vi "VCI_ReadErrInfo.vi"(8 "error in (no error)":errorcluster caption="错误输入（无错误）", 9 "CANIndex":u32, 10 "DevIndex":u32, 11 "DevType":T2=2 items=["USB-CAN"=2, "USB-CAN2"=3]) -> (0 "error out":errorcluster caption="错误输出", 2 "VCI_ERR_INFO":T1, 3 "Return Val":T3=1 items=["OK"=1, "ERROR1"=0, "ERROR2"=-1])   [LabVIEW 2018, in "ControlCan.lvlib"]
uses:
  ControlCan.lvlib
  Return Val.ctl
  DevType.ctl
  VCI_ERR_INFO.ctl
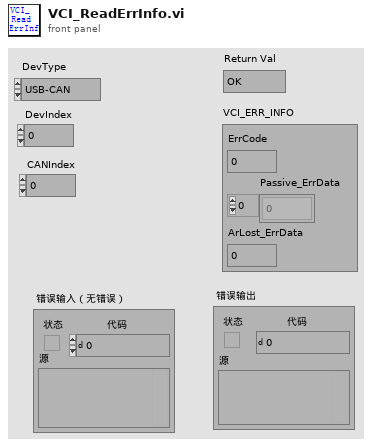
[diagram p1: front panel]
types:
  T1 = typedef "ControlCAN.lvlib/VCI_ERR_INFO.ctl" = cluster{"ErrCode":u32, "Passive_ErrData":u8[], "ArLost_ErrData":u8}
  T2 = typedef "ControlCAN.lvlib/DevType.ctl" = u32
  T3 = typedef "ControlCAN.lvlib/Return Val.ctl" = i32
  T4 = typedef "ControlCAN.lvlib/VCI_ERR_INFO_1.ctl" = cluster{"ErrCode":u32, "Passive_ErrData 0":u8, "Passive_ErrData 1":u8, "Passive_ErrData 2":u8, "ArLost_ErrData":u8}
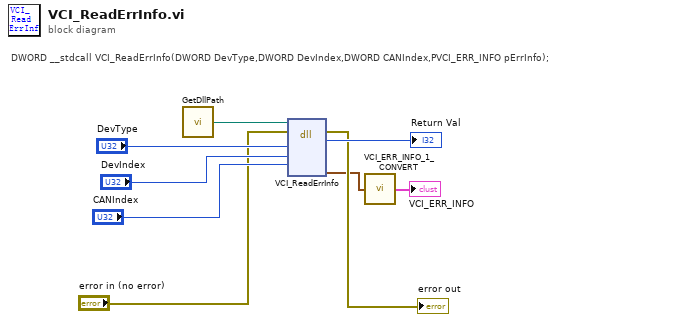
[diagram p0: block diagram]
diagram:
  # "DWORD __stdcall VCI_ReadErrInfo(DWORD DevType,DWORD DevIndex,DWORD CANIndex,PVCI_ERR_INFO pErrInfo);"
  n1 = call "GetDllPath.vi"() -> ("DllPath"=w1:path)  [unwired: 1 in]
  n2 = dll-call lib="?" fn="VCI_ReadErrInfo"(path in=w1, error in="error in (no error)", "DevType"="DevType", "DevIndex"="DevIndex", "CANIndex"="CANIndex") -> (error out=→"error out":errorcluster, "ReturnVal"=→"Return Val":i32, "VCI_ERR_INFO_1"=w3:T4)  [unwired: 5 in, 1 out]
  n3 = call "VCI_ERR_INFO_1_CONVERT.vi"("VCI_ERR_INFO_1"=w3) -> ("VCI_ERR_INFO"=→"VCI_ERR_INFO":T1)
